vi "TAT_Start.vi"(8 "error In":errorcluster) -> (0 "error out":errorcluster)   [LabVIEW 2017]
uses:
  Controls/Ass. Loop Control.ctl
  <vilib>/Utility/error.llb/DialogType.ctl
panel:
  in  "REMOVE PART":bool
  in  "ADD PART":bool
  in  "LIST OF PARTS":string(combo)
  in  "DOORS":string(combo)
  in  "DOORS":enum32{"Page 1", "Page 2"}(tab)
  out "DOOR 1":string[](array[string])
  out "DOOR 2":string[](array[string])
  out "DOOR 3":string[](array[string])
  out "DOOR 4":string[](array[string])
  out "DOOR 5":string[](array[string])
  out "DOOR 16":string[](array[string])
  out "DOOR 11":string[](array[string])
  out "DOOR 12":string[](array[string])
  out "DOOR 13":string[](array[string])
  out "DOOR 14":string[](array[string])
  out "DOOR 15":string[](array[string])
  out "USER:-":string
  in  "Stop":bool
  out "DATE/TIME":string
  out "Screen Name":string
  # "Nm"
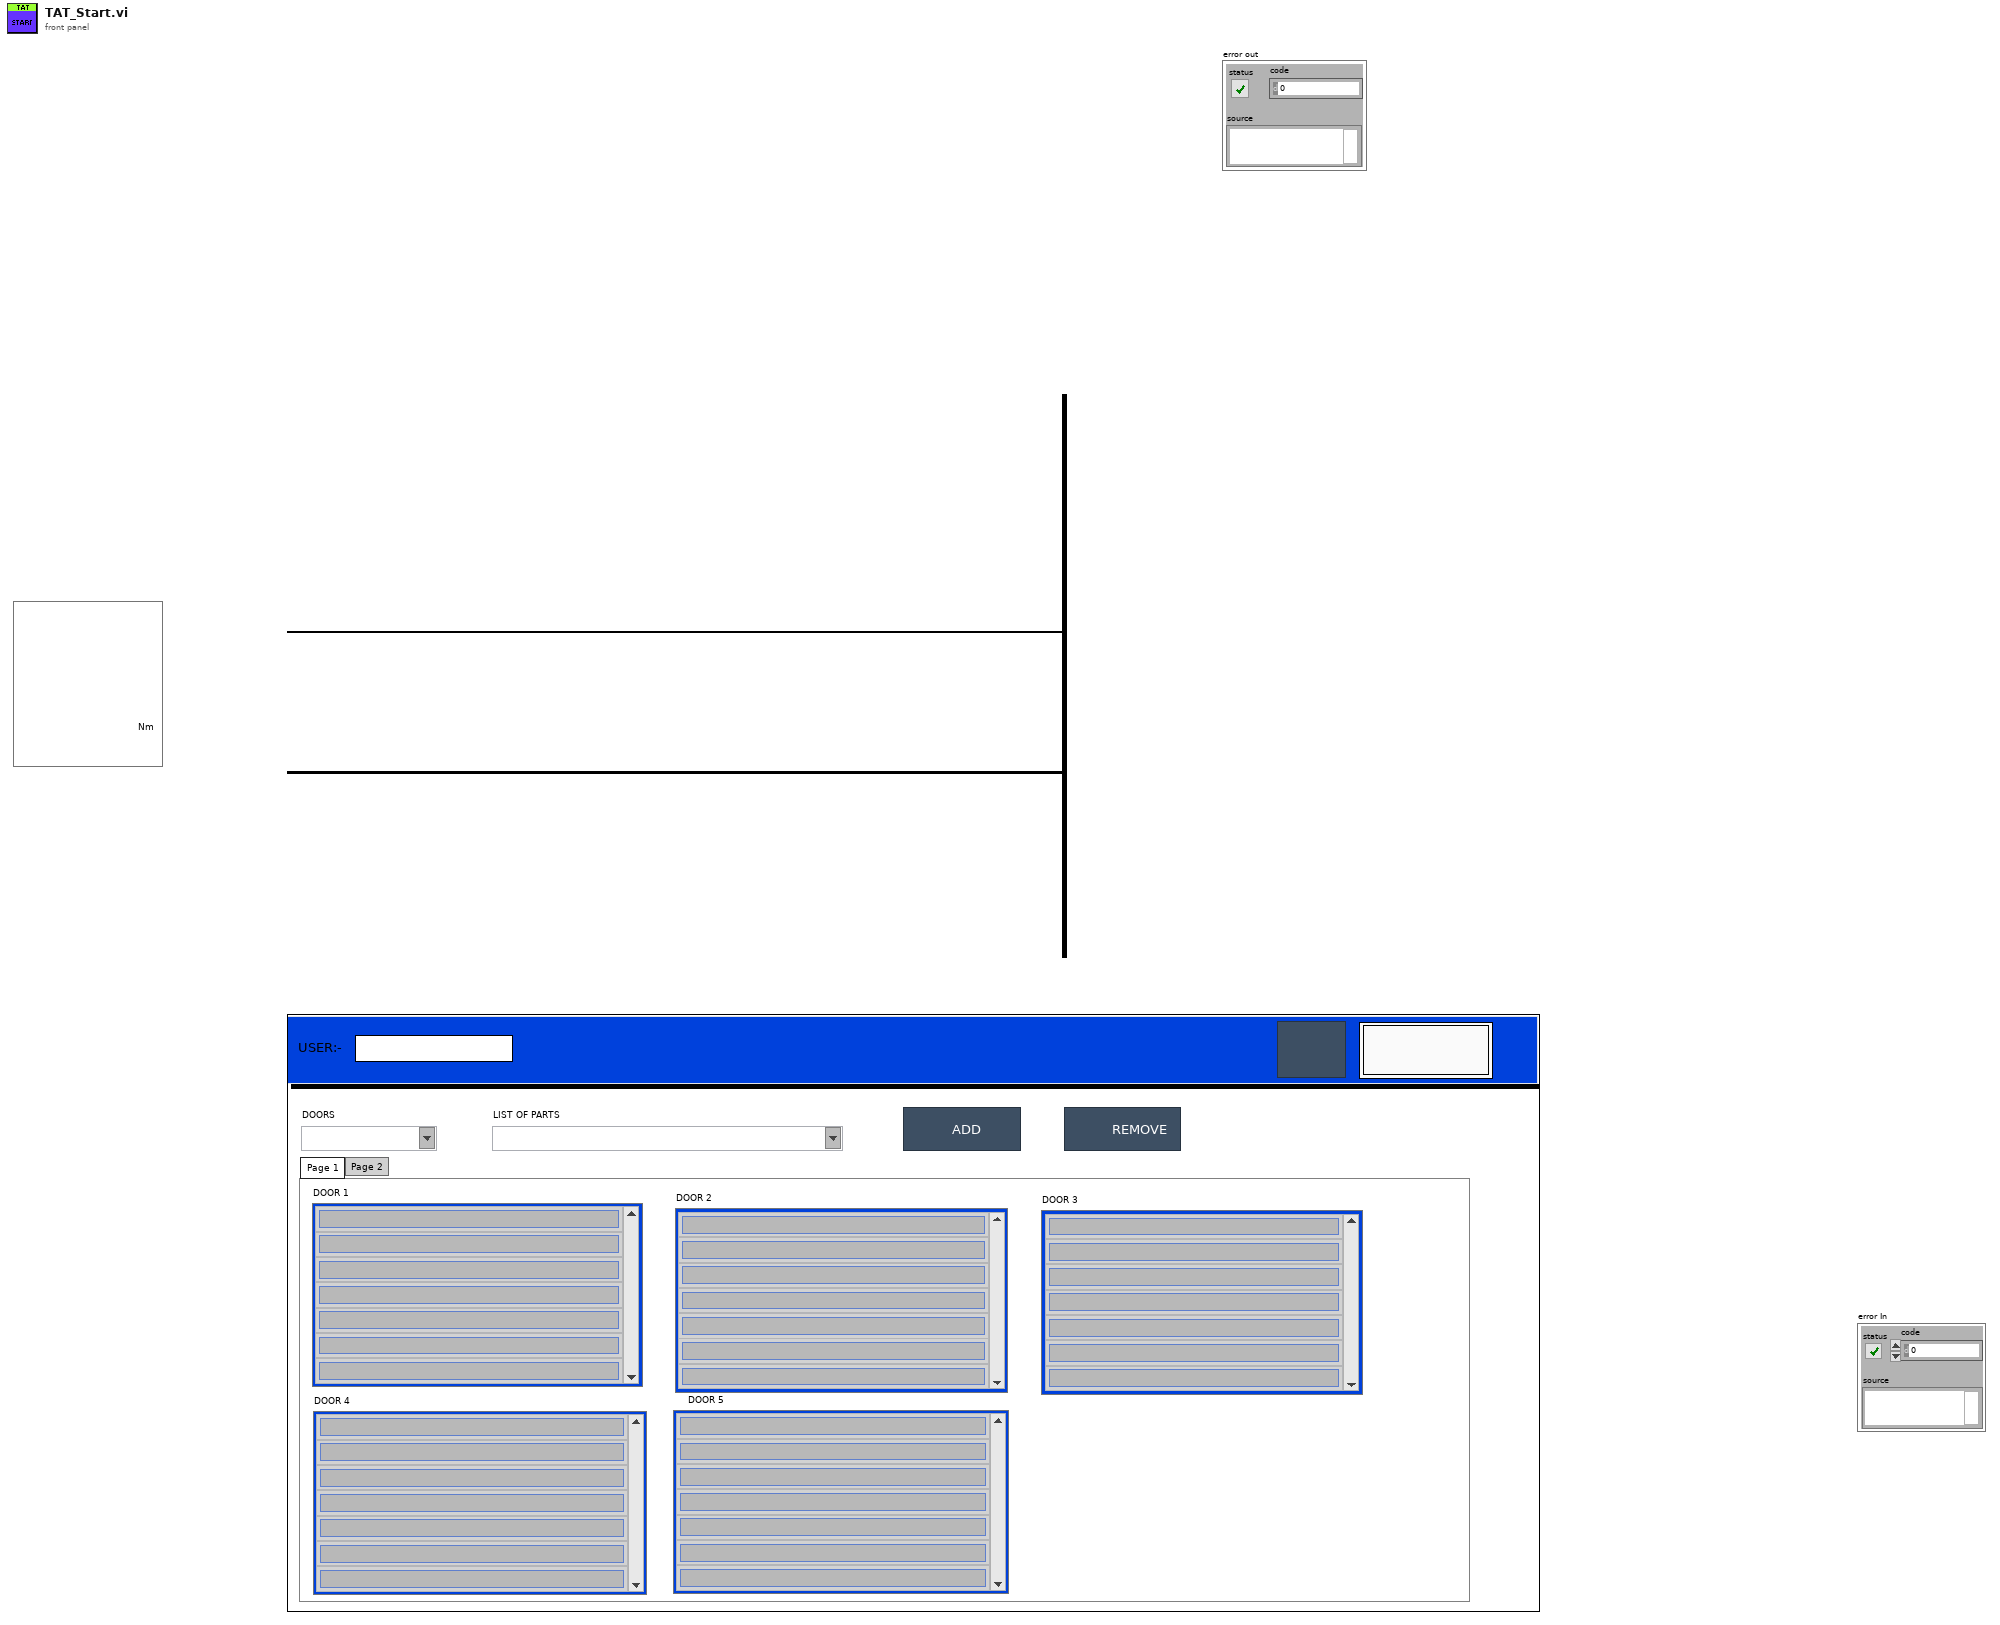
[diagram p1: front panel]
types:
  T1 = typedef "DialogType.ctl" = u16
  T2 = typedef "Ass. Loop Control.ctl" = enum16{"Package_Qty_Count", "GENERATE_QR_PRNT", "Cluster_update", "Waiting_for_scan", "barcode CHECK", "Int", "SaveReport ", "Barcode Print", "Start Cycle", "Wait", "Cycle End", "Stop"}
  T3 = enum32{"invalid app kind", "Development System", "Run Time System", "Student Edition", "Embedded LabVIEW", "Evaluation", "Custom"}
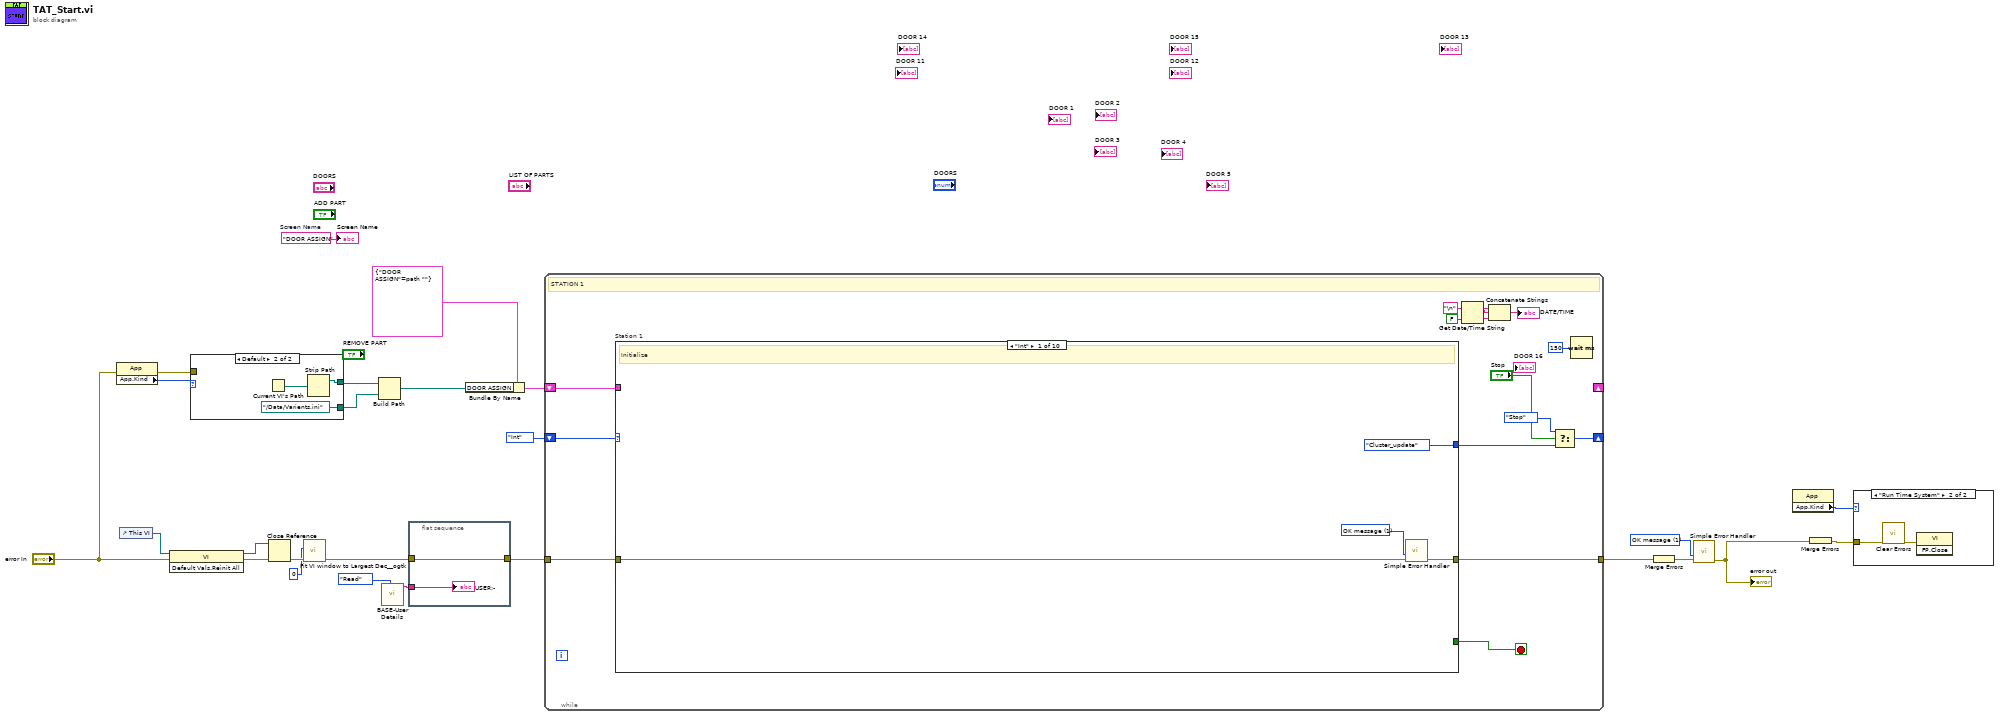
[diagram p0: block diagram]
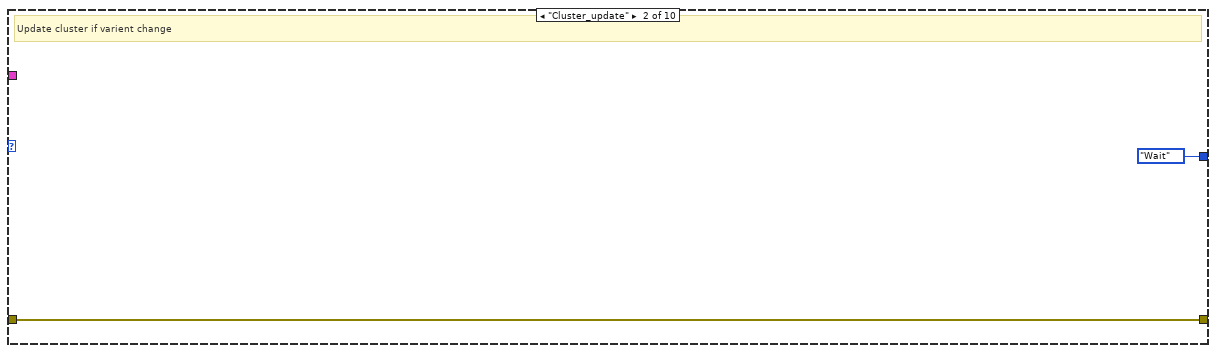
[diagram p3: hidden frame]
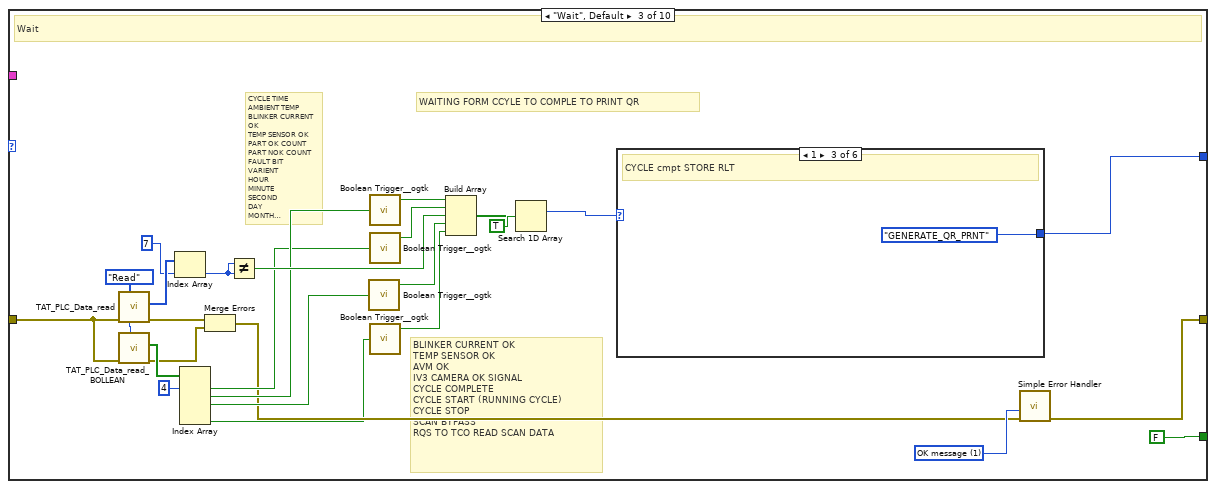
[diagram p4: hidden frame]
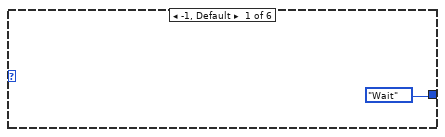
[diagram p5: hidden frame]
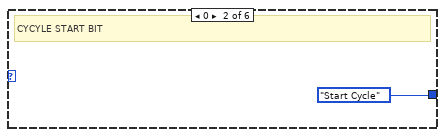
[diagram p6: hidden frame]
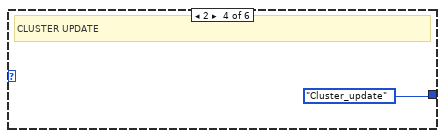
[diagram p7: hidden frame]
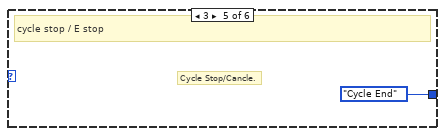
[diagram p8: hidden frame]
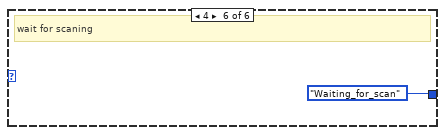
[diagram p9: hidden frame]
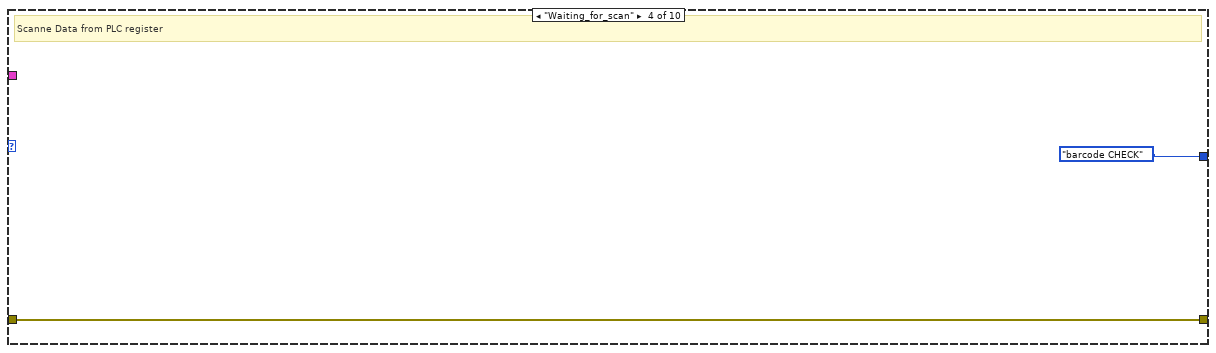
[diagram p10: hidden frame]
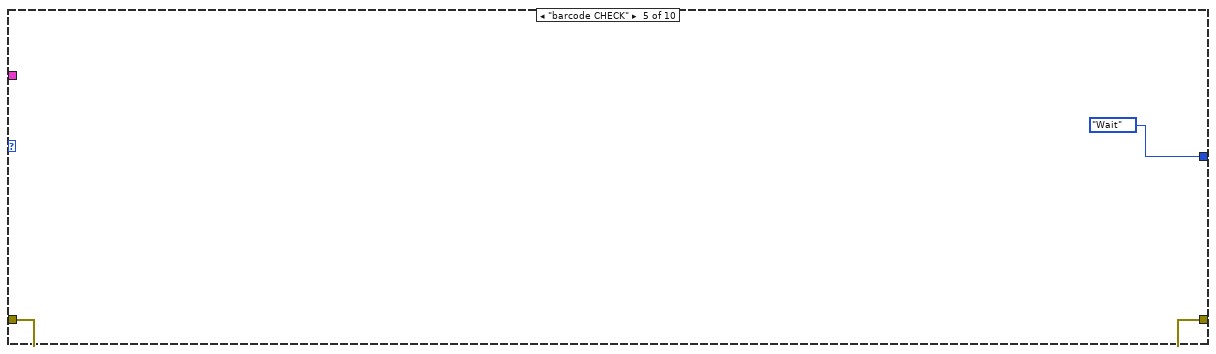
[diagram p11: hidden frame]
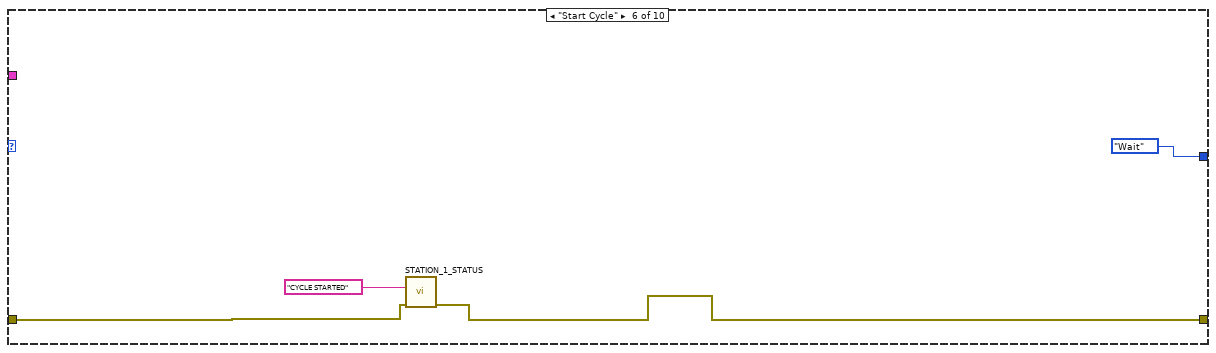
[diagram p12: hidden frame]
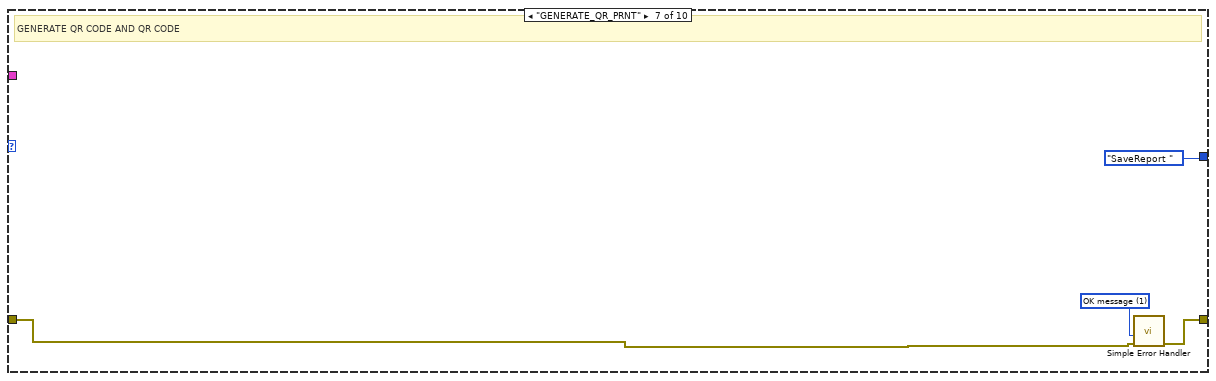
[diagram p13: hidden frame]
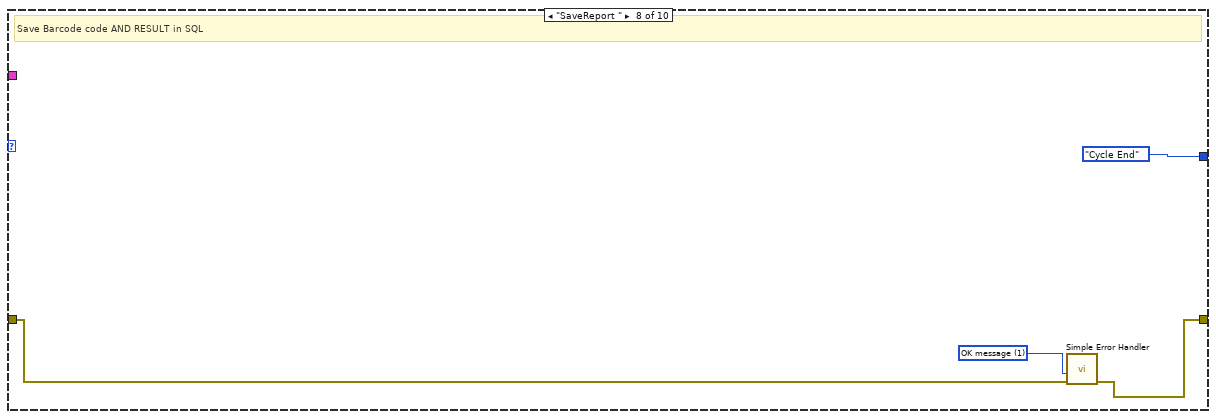
[diagram p14: hidden frame]
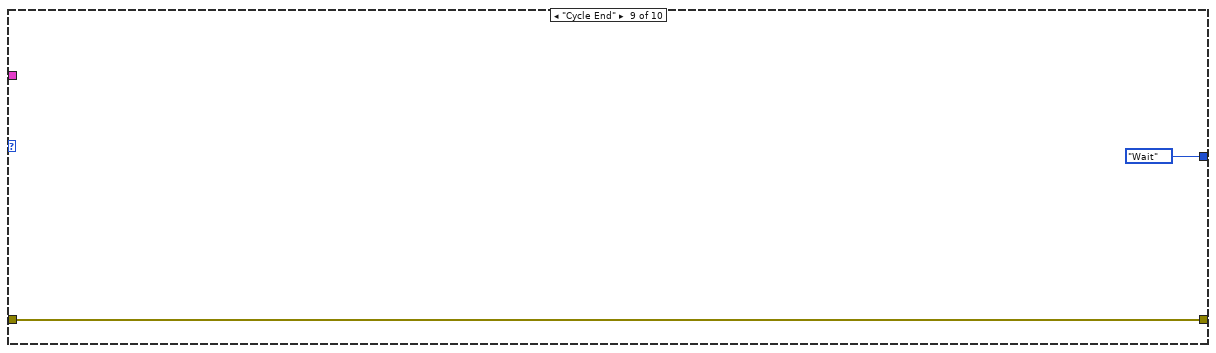
[diagram p15: hidden frame]
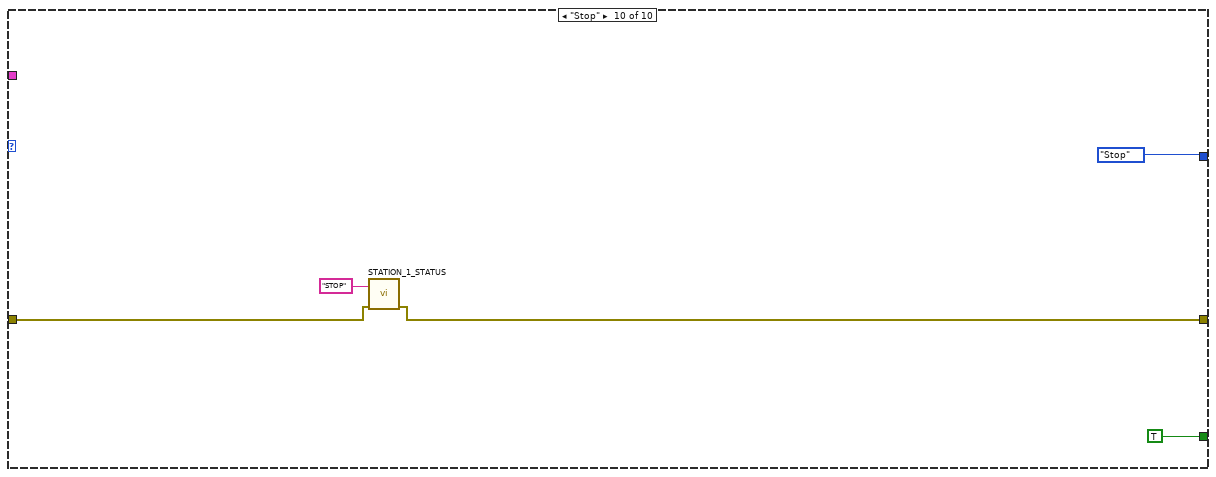
[diagram p16: hidden frame]
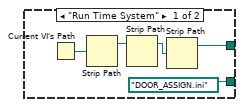
[diagram p17: hidden frame]
diagram:
  w4 = "DOOR ASSIGN"  # Screen Name
  w16 = T1 1 items=["no dialog", "OK message", "continue or stop message", "OK message + warnings", "continue/stop + warnings"] ("type of dialog (OK msg:1)")
  n1 = property class="App"(error in="error In") -> (error out=w12:errorcluster, "App.Kind"=w14:T3)  [unwired: 1 in, 1 out]
  n2 = control-ref of="This VI"() -> (w25:refnum<vi>)
  n3 = invoke class="VI" method="Default Vals.Reinit All"(reference=w25, error in="error In") -> (reference out=w23:refnum<vi>, error out=w24:errorcluster)  [unwired: 1 in, 1 out]
  n4 = case shown="Default" w14 {
    tunnel: [path "DOOR_ASSIGN.ini" ("path") path "../Data/Varients.ini" ("path")] -> w13
    tunnel: [w26 w31] -> w6
    tunnel: w12 -> [_ _]
    frame "Run Time System" {
      n5 = Current VI's Path() -> (path=w29:path)
      n6 = Strip Path(path=w29) -> (stripped path=w28:path)  [unwired: 1 out]
      n7 = Strip Path(path=w28) -> (stripped path=w27:path)  [unwired: 1 out]
      n8 = Strip Path(path=w27) -> (stripped path=w26:path)  [unwired: 1 out]
    }
    frame Default {
      n9 = Current VI's Path() -> (path=w32:path)
      n10 = Strip Path(path=w32) -> (stripped path=w31:path)  [unwired: 1 out]
    }
  }
  n11 = Close Reference(reference=w23, error in (no error)=w24) -> (error out=w22:errorcluster)
  n12 = call <userlib>:"Fit VI window to Largest Dec__ogtk.vi"("error in (no error)"=w22, "border spacing (2 px)"=0) -> ("error out"=w10:errorcluster)  [unwired: 4 in, 1 out]
  n13 = Build Path(base path=w6, name or relative path=w13) -> (appended path=w2:path)
  n14 = call "BASE-User Details.vi"("Enum"=enum16{"Read", "Write"}."Read") -> ("User Name Out"=w17:string)  [unwired: 9 in, 1 out]
  n15 = flat-sequence {
    tunnel: [w35] -> w5
    tunnel: w10 -> [w35]
    tunnel: w17 -> [w34]
    frame #0 {
      "USER:-" <- w34
    }
  }
  n16 = Bundle By Name(cluster=cluster{"DOOR ASSIGN":path} {"DOOR ASSIGN"=path ""}, "DOOR ASSIGN"=w2) -> (w1:cluster{"DOOR ASSIGN":path})
  n17 = while {
    tunnel: w5 -> [w37]
    shift-right: [w47] -> _
    shift-left: Ass._Loop_Control."Int" ("Enum") -> [w50]
    tunnel: [w48] -> w20
    shift-right: _ -> [_]
    shift-left: w1 -> [w36]
    stop <- w40 stop-if-true
    # "STATION 1"
    n18 = case "Station 1" shown="\"Int\"" w50 {
      tunnel: [Ass._Loop_Control."Cluster_update" ("Enum") Ass._Loop_Control."Wait" ("Enum") w76 Ass._Loop_Control."barcode CHECK" ("Enum") Ass._Loop_Control."Wait" ("Enum") Ass._Loop_Control."Wait" ("Enum") Ass._Loop_Control."SaveReport " ("Enum") Ass._Loop_Control."Cycle End" ("Enum") Ass._Loop_Control."Wait" ("Enum") Ass._Loop_Control."Stop" ("Enum")] -> w39
      tunnel: [_ _ FALSE _ _ _ _ _ _ TRUE] -> w40
      tunnel: [w52 w55 w73 w89 w91 w93 w99 w102 w105 w107] -> w48
      tunnel: w37 -> [w51 w55 w70 w89 w91 w94 w97 w101 w105 w108]
      tunnel: w36 -> [_ _ _ _ _ _ _ _ _ _]
      frame "Int" {
        w53 = T1 1 items=["no dialog", "OK message", "continue or stop message", "OK message + warnings", "continue/stop + warnings"] ("type of dialog (OK msg:1)")
        # "Initialize"
        n19 = call <vilib>:"Simple Error Handler.vi"("type of dialog (OK msg:1)"=w53, "error in (no error)"=w51) -> ("error out"=w52:errorcluster)  [unwired: 3 in, 4 out]
      }
      frame "Cluster_update" {
        # "Update cluster if varient change"
      }
      frame "Wait", Default {
        w74 = T1 1 items=["no dialog", "OK message", "continue or stop message", "OK message + warnings", "continue/stop + warnings"] ("type of dialog (OK msg:1)")
        w71 = enum16{"Read", "Write"}."Read" ("Enum")
        # "CYCLE TIME\nAMBIENT TEMP\nBLINKER CURRENT OK\nTEMP SENSOR OK\nPART OK COUNT\nPART NOK COUNT\nFAULT BIT\nVARIENT\nHOUR\nMINUTE\nSECOND\nDAY\nMONTH\nYEAR\nSERIAL NUMBER"
        # "BLINKER CURRENT OK\nTEMP SENSOR OK\nAVM OK\nIV3 CAMERA OK SIGNAL\nCYCLE COMPLETE\nCYCLE START (RUNNING CYCLE)\nCYCLE STOP\nSCAN BYPASS\nRQS TO TCO READ SCAN DATA"
        # "WAITING FORM CCYLE TO COMPLE TO PRINT QR"
        # "Wait"
        n20 = call "TAT_PLC_Data_read.vi"("Enum"=w71, "error in (no error)"=w70) -> ("error out"=w61:errorcluster, "Array 2"=w77:u16[])  [unwired: 8 in]
        n21 = call "TAT_PLC_Data_read_BOLLEAN.vi"("Enum"=w71, "error in (no error)"=w70) -> ("error out"=w59:errorcluster, "Array 2"=w69:bool[])  [unwired: 8 in]
        n22 = Index Array(array=w77, index=7) -> (element=w57:u16)
        n23 = Index Array(array=w69, index #1=4 ("index")) -> (element #1=w66:bool, element #2=w67:bool, element #3=w65:bool, element #5=w58:bool)  [unwired: 4 in, 1 out]
        n24 = Merge Errors(w61, w59) -> (w60:errorcluster)
        n25 = Not Equal?(x=w57, y=w57) -> (x != y?=w75:bool)
        n26 = call <userlib>:"Boolean Trigger__ogtk.vi"("Boolean Input"=w65) -> ("Rising Edge"=w64:bool)  [unwired: 1 in, 1 out]
        n27 = call <userlib>:"Boolean Trigger__ogtk.vi"("Boolean Input"=w67) -> ("Rising Edge"=w81:bool)  [unwired: 1 in, 1 out]
        n28 = call <userlib>:"Boolean Trigger__ogtk.vi"("Boolean Input"=w66) -> ("Rising Edge"=w72:bool)  [unwired: 1 in, 1 out]
        n29 = call <userlib>:"Boolean Trigger__ogtk.vi"("Boolean Input"=w58) -> ("Rising Edge"=w63:bool)  [unwired: 1 in, 1 out]
        n30 = Build Array(w81, w72, w75, w64, w63) -> (w80:bool[])
        n31 = Search 1D Array(1D array=w80, element=TRUE ("Boolean Input")) -> (index of element=w79:i32)  [unwired: 1 in]
        n32 = case shown="1" w79 {
          tunnel: [Ass._Loop_Control."Wait" ("Enum") Ass._Loop_Control."Start Cycle" ("Enum") Ass._Loop_Control."GENERATE_QR_PRNT" ("Enum") Ass._Loop_Control."Cluster_update" ("Enum") Ass._Loop_Control."Cycle End" ("Enum") Ass._Loop_Control."Waiting_for_scan" ("Enum")] -> w76
          frame -1, Default {
          }
          frame 0 {
            # "CYCYLE START BIT"
          }
          frame 1 {
            # "CYCLE cmpt STORE RLT"
          }
          frame 2 {
            # "CLUSTER UPDATE"
          }
          frame 3 {
            # "Cycle Stop/Cancle."
            # "cycle stop / E stop"
          }
          frame 4 {
            # "wait for scaning"
          }
        }
        n33 = call <vilib>:"Simple Error Handler.vi"("type of dialog (OK msg:1)"=w74, "error in (no error)"=w60) -> ("error out"=w73:errorcluster)  [unwired: 3 in, 4 out]
      }
      frame "Waiting_for_scan" {
        # "Scanne Data from PLC register"
      }
      frame "barcode CHECK" {
      }
      frame "Start Cycle" {
        n34 = call "STATION_1_STATUS.vi"("error in (no error)"=w94, "STATUS"="CYCLE STARTED" ("Cycle Status")) -> ("error out"=w93:errorcluster)  [unwired: 9 in]
      }
      frame "GENERATE_QR_PRNT" {
        w100 = T1 1 items=["no dialog", "OK message", "continue or stop message", "OK message + warnings", "continue/stop + warnings"] ("type of dialog (OK msg:1)")
        # "GENERATE QR CODE AND QR CODE"
        n35 = call <vilib>:"Simple Error Handler.vi"("type of dialog (OK msg:1)"=w100, "error in (no error)"=w97) -> ("error out"=w99:errorcluster)  [unwired: 3 in, 4 out]
      }
      frame "SaveReport " {
        w103 = T1 1 items=["no dialog", "OK message", "continue or stop message", "OK message + warnings", "continue/stop + warnings"] ("type of dialog (OK msg:1)")
        # "Save Barcode code AND RESULT in SQL"
        n36 = call <vilib>:"Simple Error Handler.vi"("type of dialog (OK msg:1)"=w103, "error in (no error)"=w101) -> ("error out"=w102:errorcluster)  [unwired: 3 in, 4 out]
      }
      frame "Cycle End" {
      }
      frame "Stop" {
        n37 = call "STATION_1_STATUS.vi"("error in (no error)"=w108, "STATUS"="STOP" ("Cycle Status")) -> ("error out"=w107:errorcluster)  [unwired: 9 in]
      }
    }
    n38 = Get Date/Time String(want seconds? (F)=FALSE) -> (date string=w44:string, time string=w43:string)  [unwired: 2 in]
    n39 = Concatenate Strings(w44, "\n", w43) -> (→"DATE/TIME":string)
    n40 = Select(t=Ass._Loop_Control."Stop" ("Enum"), s="Stop", f=w39) -> (s? t:f=w47:T2)
    n41 = Wait (ms)(milliseconds to wait=u32 150) -> ()  [unwired: 1 out]
  }
  n42 = Merge Errors(w20) -> (w19:errorcluster)
  n43 = call <vilib>:"Simple Error Handler.vi"("type of dialog (OK msg:1)"=w16, "error in (no error)"=w19) -> ("error out"=w7:errorcluster)  [unwired: 3 in, 4 out]
  "error out" <- w7
  n44 = property class="App"() -> ("App.Kind"=w15:T3)  [unwired: 2 in, 2 out]
  n45 = Merge Errors(w7) -> (w8:errorcluster)
  n46 = case shown="\"Run Time System\"" w15 {
    tunnel: w8 -> [_ w113]
    frame "invalid app kind", Default {
    }
    frame "Run Time System" {
      n47 = call <vilib>:"Clear Errors.vi"("error in (no error)"=w113) -> ("error out"=w112:errorcluster)  [unwired: 5 in, 1 out]
      n48 = invoke class="VI" method="FP.Close"(error in=w112) -> ()  [unwired: 2 in, 3 out]
    }
  }
  "Screen Name" <- w4
